vi "Matlab-Calc.vi"(0 "Temp-Array":dbl[](array[numeric]), 3 "Matlab?":bool, 4 "Leistung":dbl, 6 "Druck-Array":dbl[](array[numeric]), 10 "FI Öl":dbl) -> (7 "TI08_neu":dbl, 8 "Dampfkonzentration":dbl, 9 "m_reich [g/s]":dbl, 11 "Konzentration_reich":dbl, 12 "Dif-Siedetemperatur":dbl, 13 "m_arm [g/s]":dbl, 14 "Dampfmassenstrom [g/s]":dbl, 15 "Dichte_reich [kg/m³]":dbl, 16 "Siedetemperatur":dbl, 17 "Dampfmassenanteil":dbl, 18 "m_vap [kg/s]":dbl, 19 "v_vap [l/min]":dbl)   [LabVIEW 2015]
panel:
  out "xi_r":dbl format="%#_13g"
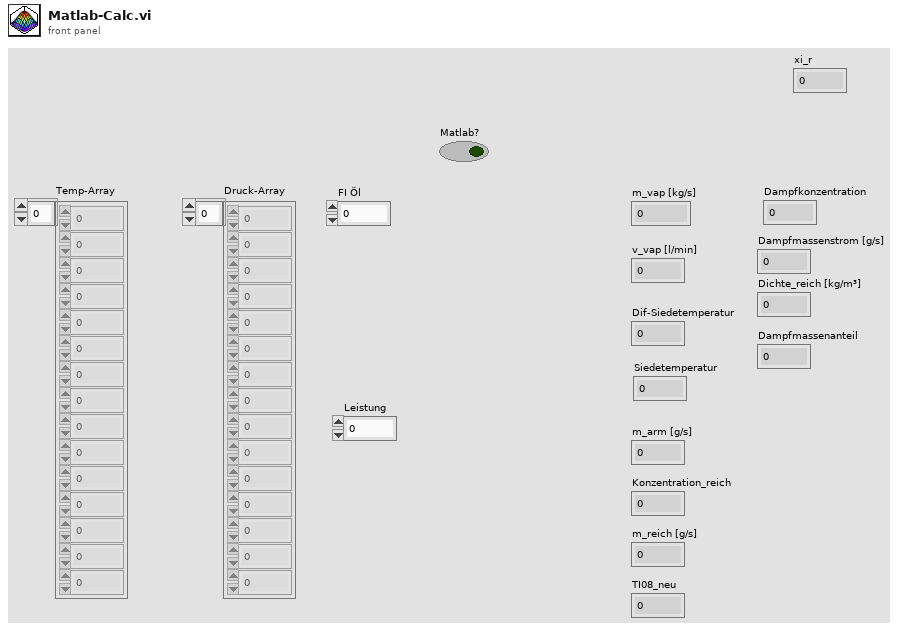
[diagram p1: front panel]
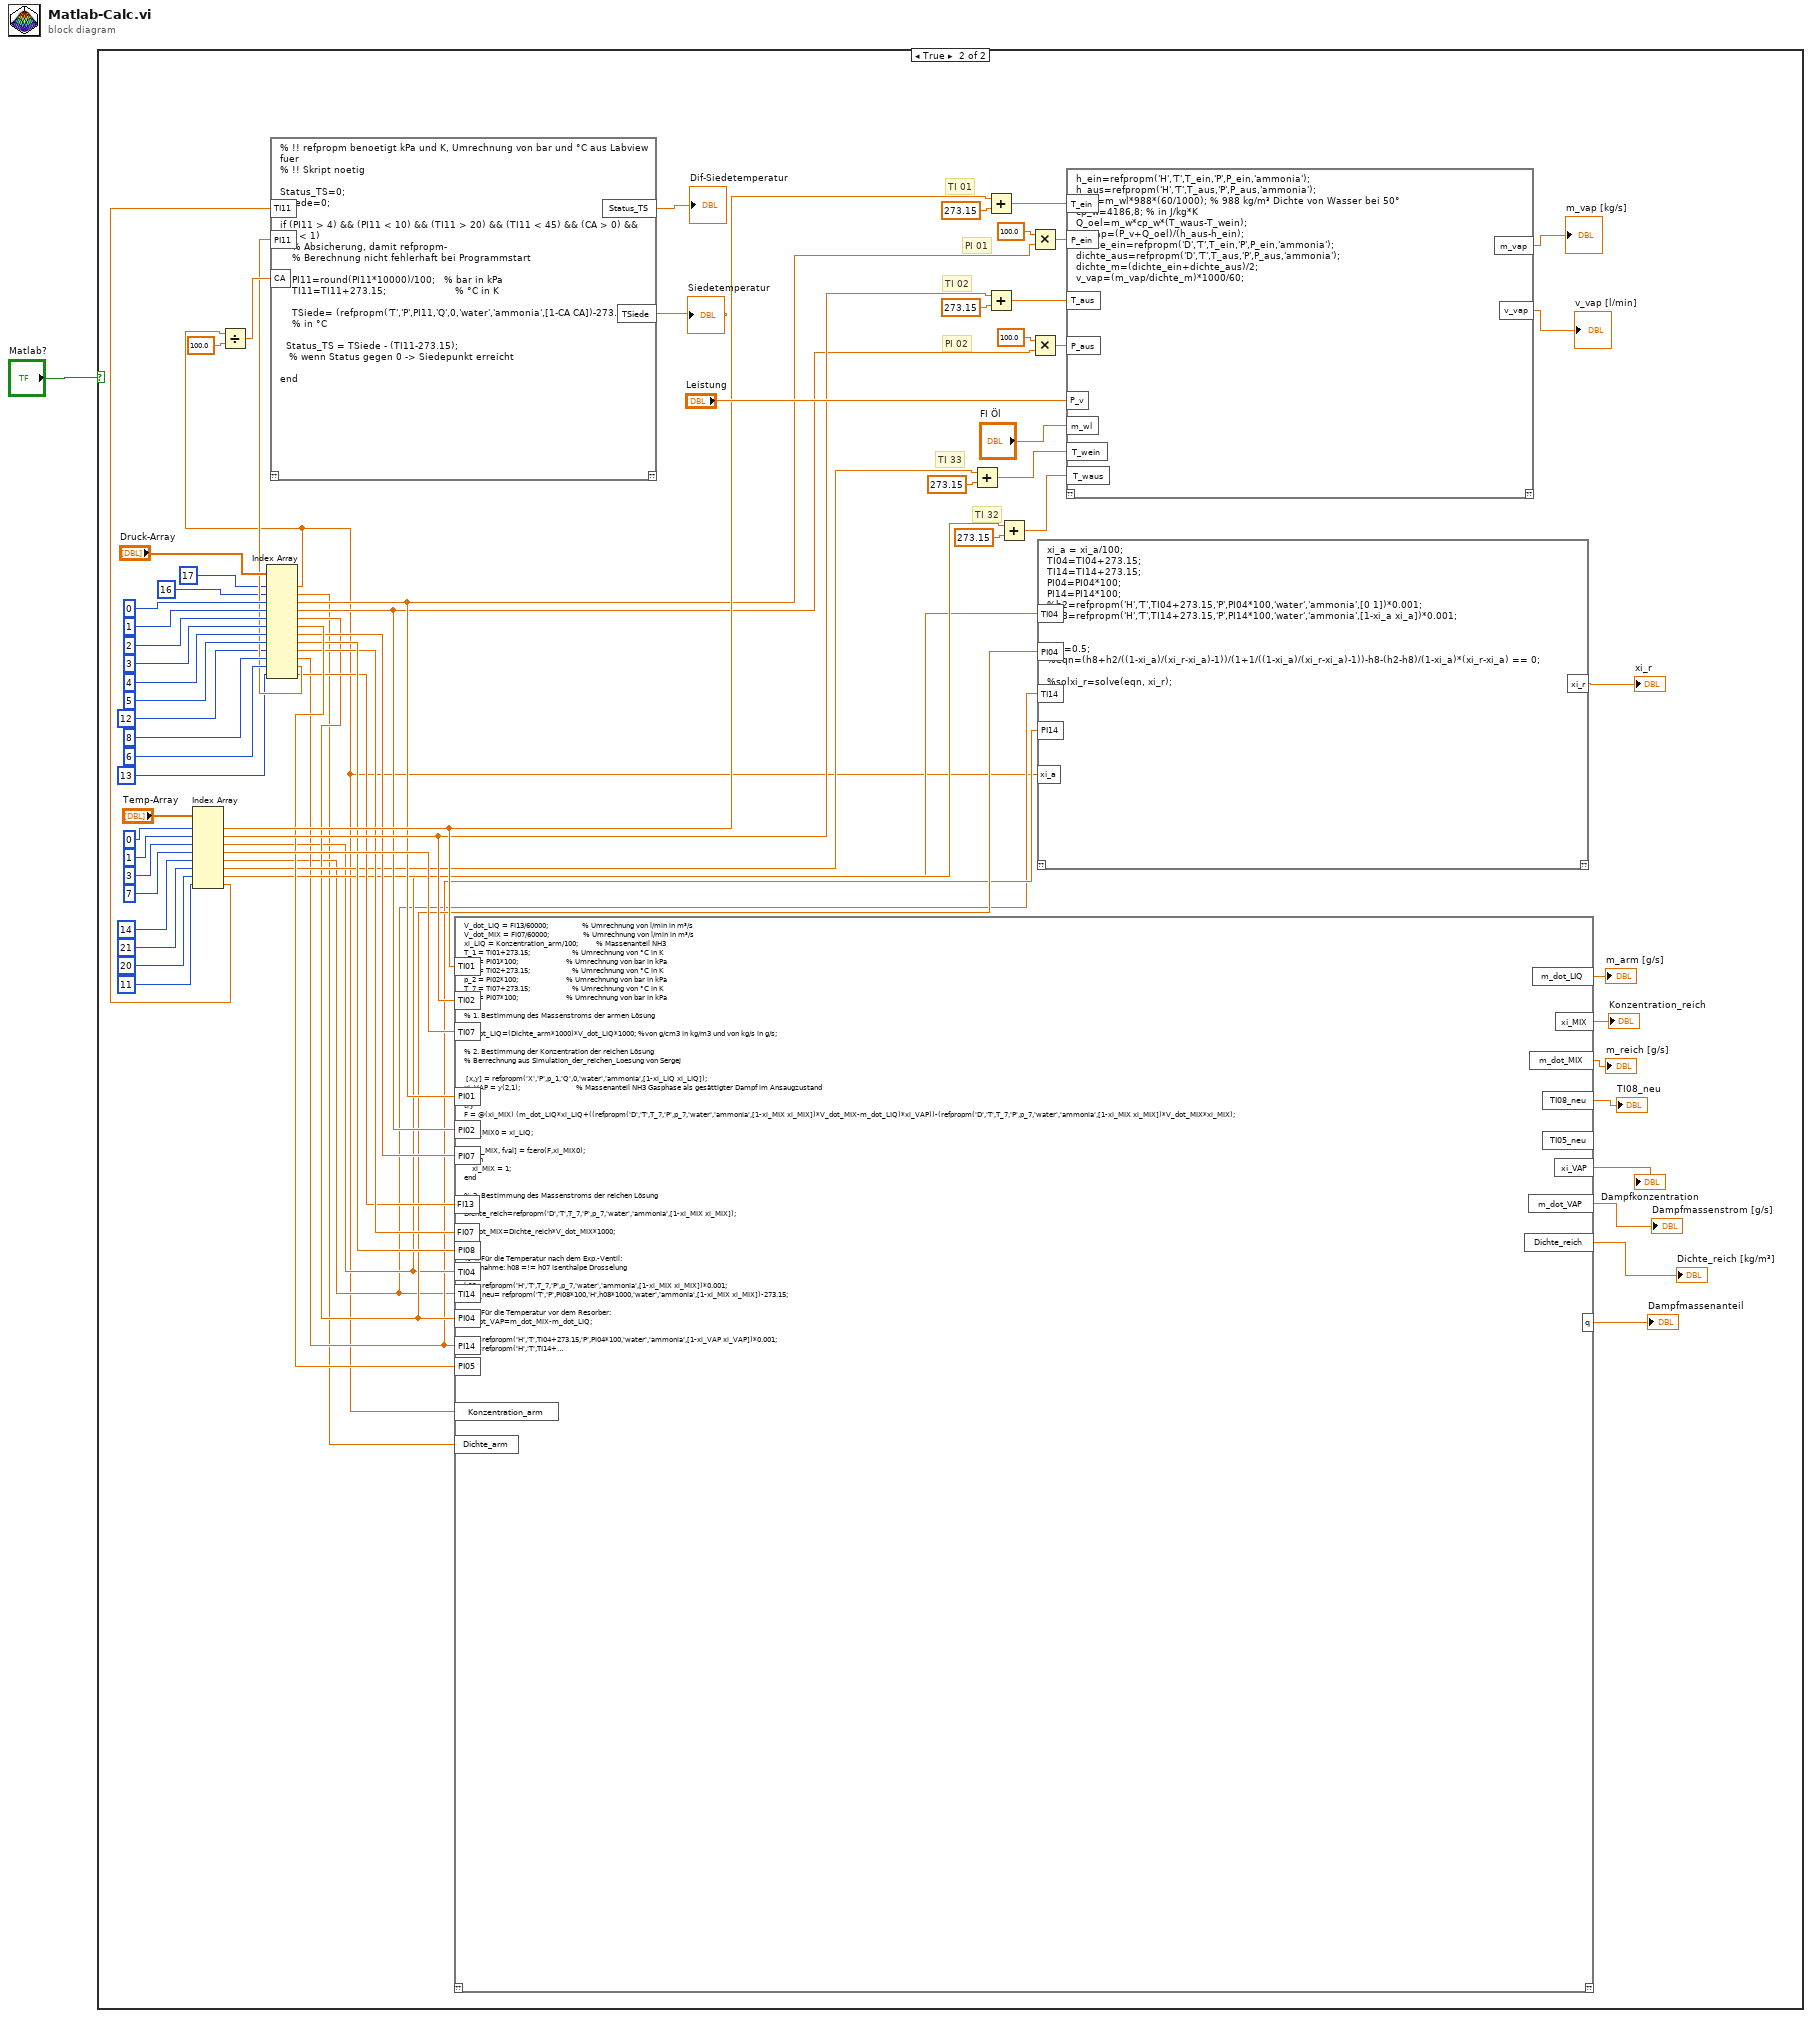
[diagram p0: block diagram]
diagram:
  n1 = case shown="True" "Matlab?" {
    frame False {
    }
    frame True {
      # "TI 02"
      # "TI 01"
      # "TI 32"
      # "TI 33"
      # "PI 02"
      # "PI 01"
      n2 = Index Array(array="Temp-Array", index #1=0 ("index"), index #2=1 ("index"), index #3=3 ("index"), index #4=7 ("index"), index #5=14 ("index"), index #6=21 ("index"), index #7=20 ("index"), index #8=11 ("index")) -> (element #1=w47:dbl, element #2=w46:dbl, element #3=w9:dbl, element #4=w49:dbl, element #5=w7:dbl, element #6=w13:dbl, element #7=w12:dbl, element #8=w11:dbl)
      n3 = Index Array(array="Druck-Array", index #1=17 ("index"), index #2=16 ("index"), index #3=0 ("index"), index #4=1 ("index"), index #5=2 ("index"), index #6=3 ("index"), index #7=4 ("index"), index #8=5 ("index"), index #9=12 ("index"), index #10=8 ("index"), index #11=6 ("index"), index #12=13 ("index")) -> (element #1=w2:dbl, element #2=w4:dbl, element #3=w34:dbl, element #4=w33:dbl, element #5=w10:dbl, element #6=w38:dbl, element #7=w37:dbl, element #8=w36:dbl, element #9=w19:dbl, element #10=w8:dbl, element #11=w35:dbl, element #12=w18:dbl)
      n4 = Divide(x=w2, y=100.0) -> (x/y=w70:dbl)
      n5 = script code="% !! refpropm benoetigt kPa und K, Umrechnung von bar und °C aus Labview fuer\n% !! Skript noetig\n\nStatus_TS=0;\nTSiede=0;\n\nif (PI11 > 4) && (PI11 < 10) && (TI11 > 20) && (TI11 < 45) && (CA > 0) && (CA < 1)     \n    % Absicherung, damit refpropm-   \n    % Berechnung nicht fehlerhaft bei Programmstart    \n    \n    PI11=round(PI11*10000)/100;   % bar in kPa\n    TI11=TI11+273.15;                       % °C in K  \n        \n    TSiede= (refpropm('T','P',PI11,'Q',0,'water','ammonia',[1-CA CA])-273.15);\n    % in °C\n    \n  Status_TS = TSiede - (TI11-273.15);\n   % wenn Status gegen 0 -> Siedepunkt erreicht \n    \nend"("TI11"=w11, "PI11"=w35, "CA"=w70) -> ("Status_TS"=→"Dif-Siedetemperatur":dbl, "TSiede"=→"Siedetemperatur":dbl)  [unwired: 1 in, 1 out]
      n6 = script code="V_dot_LIQ = FI13/60000;                 % Umrechnung von l/min in m³/s\nV_dot_MIX = FI07/60000;                 % Umrechnung von l/min in m³/s\nxi_LIQ = Konzentration_arm/100;         % Massenanteil NH3                      \nT_1 = TI01+273.15;                     % Umrechnung von °C in K\np_1 = PI01*100;                        % Umrechnung von bar in kPa\nT_2 = TI02+273.15;                     % Umrechnung von °C in K\np_2 = PI02*100;                        % Umrechnung von bar in kPa\nT_7 = TI07+273.15;                     % Umrechnung von °C in K\np_7 = PI07*100;                        % Umrechnung von bar in kPa\n\n% 1. Bestimmung des Massenstroms der armen Lösung\n\nm_dot_LIQ=(Dichte_arm*1000)*V_dot_LIQ*1000; %von g/cm3 in kg/m3 und von kg/s in g/s;\n\n% 2. Bestimmung der Konzentration der reichen Lösung \n% Berrechnung aus Simulation_der_reichen_Loesung von Sergej\n\n [x,y] = refpropm('X','P',p_1,'Q',0,'water','ammonia',[1-xi_LIQ xi_LIQ]);\nxi_VAP = y(2,1);                            % Massenanteil NH3 Gasphase als gesättigter Dampf im Ansaugzustand\n\ntry \nF = @(xi_MIX) (m_dot_LIQ*xi_LIQ+((refpropm('D','T',T_7,'P',p_7,'water','ammonia',[1-xi_MIX xi_MIX])*V_dot_MIX-m_dot_LIQ)*xi_VAP))-(refpropm('D','T',T_7,'P',p_7,'water','ammonia',[1-xi_MIX xi_MIX])*V_dot_MIX*xi_MIX);\n\n    xi_MIX0 = xi_LIQ;\n\n    [xi_MIX, fval] = fzero(F,xi_MIX0);\ncatch\n    xi_MIX = 1;\nend\n\n% 3. Bestimmung des Massenstroms der reichen Lösung \n\nDichte_reich=refpropm('D','T',T_7,'P',p_7,'water','ammonia',[1-xi_MIX xi_MIX]);\n\nm_dot_MIX=Dichte_reich*V_dot_MIX*1000; \n\ntry\n% 4. Für die Temperatur nach dem Exp.-Ventil:\n%Annahme: h08 =!= h07 isenthalpe Drosselung\n\nh08=refpropm('H','T',T_7,'P',p_7,'water','ammonia',[1-xi_MIX xi_MIX])*0.001;\nTI08_neu= refpropm('T','P',PI08*100,'H',h08*1000,'water','ammonia',[1-xi_MIX xi_MIX])-273.15;\n\n% 5. Für die Temperatur vor dem Resorber:\nm_dot_VAP=m_dot_MIX-m_dot_LIQ;\n\nh04=refpropm('H','T',TI04+273.15,'P',PI04*100,'water','ammonia',[1-xi_VAP xi_VAP])*0.001; \nh14=refpropm('H','T',TI14+273.15,'P',PI14*100,'water','ammonia',[1-xi_LIQ xi_LIQ])*0.001;\nh05=((m_dot_LIQ*h14)+(m_dot_VAP*h04))/m_dot_MIX;\n\ncatch\nend\n\ntry\nTI05_neu=refpropm('T','P',PI05*100,'H',h05*1000,'water','ammonia',[1-xi_MIX xi_MIX])-273.15;\ncatch\nTI05_neu = 0;\nend\n\n% Dampfmassenanteil\n\nq = m_dot_VAP / m_dot_MIX;"("TI01"=w47, "TI02"=w46, "TI07"=w49, "PI01"=w34, "PI02"=w33, "PI07"=w37, "FI13"=w18, "FI07"=w19, "Konzentration_arm"=w2, "PI08"=w36, "TI04"=w9, "TI14"=w7, "PI04"=w10, "PI14"=w8, "PI05"=w38, "Dichte_arm"=w4) -> ("m_dot_LIQ"=→"m_arm [g/s]":dbl, "xi_MIX"=→"Konzentration_reich":dbl, "m_dot_MIX"=→"m_reich [g/s]":dbl, "TI08_neu"=→"TI08_neu":dbl, "xi_VAP"=→"Dampfkonzentration":dbl, "m_dot_VAP"=→"Dampfmassenstrom [g/s]":dbl, "Dichte_reich"=→"Dichte_reich [kg/m³]":dbl, "q"=→"Dampfmassenanteil":dbl)  [unwired: 1 in, 2 out]
      n7 = Add(x=w13, y=273.15) -> (x+y=w56:dbl)
      n8 = Add(x=w47, y=273.15) -> (x+y=w66:dbl)
      n9 = Add(x=w46, y=273.15) -> (x+y=w67:dbl)
      n10 = Add(x=w12, y=273.15) -> (x+y=w55:dbl)
      n11 = Multiply(x=100.0, y=w34) -> (x*y=w61:dbl)
      n12 = Multiply(x=100.0, y=w33) -> (x*y=w63:dbl)
      n13 = script code="xi_a = xi_a/100;\nTI04=TI04+273.15;\nTI14=TI14+273.15;\nPI04=PI04*100;\nPI14=PI14*100;\n%h2=refpropm('H','T',TI04+273.15,'P',PI04*100,'water','ammonia',[0 1])*0.001; \n%h8=refpropm('H','T',TI14+273.15,'P',PI14*100,'water','ammonia',[1-xi_a xi_a])*0.001;\n\n\nxi_r=0.5;\n%eqn=(h8+h2/((1-xi_a)/(xi_r-xi_a)-1))/(1+1/((1-xi_a)/(xi_r-xi_a)-1))-h8-(h2-h8)/(1-xi_a)*(xi_r-xi_a) == 0;\n\n%solxi_r=solve(eqn, xi_r);"("TI04"=w9, "PI04"=w10, "TI14"=w7, "PI14"=w8, "xi_a"=w2) -> ("xi_r"=→"xi_r":dbl)  [unwired: 1 in, 1 out]
      n14 = script code="h_ein=refpropm('H','T',T_ein,'P',P_ein,'ammonia');\nh_aus=refpropm('H','T',T_aus,'P',P_aus,'ammonia');\nm_w=m_wl*988*(60/1000); % 988 kg/m³ Dichte von Wasser bei 50° \ncp_w=4186,8; % in J/kg*K \nQ_oel=m_w*cp_w*(T_waus-T_wein);\nm_vap=(P_v+Q_oel)/(h_aus-h_ein);\ndichte_ein=refpropm('D','T',T_ein,'P',P_ein,'ammonia');\ndichte_aus=refpropm('D','T',T_aus,'P',P_aus,'ammonia');\ndichte_m=(dichte_ein+dichte_aus)/2;\nv_vap=(m_vap/dichte_m)*1000/60;"("T_ein"=w66, "P_ein"=w61, "T_aus"=w67, "P_aus"=w63, "P_v"="Leistung", "m_wl"="FI Öl", "T_wein"=w56, "T_waus"=w55) -> ("m_vap"=→"m_vap [kg/s]":dbl, "v_vap"=→"v_vap [l/min]":dbl)  [unwired: 1 in, 1 out]
    }
  }
